vi "Transition State.vi"(8 "Error In":errorcluster, 10 "L       E \nIndicator":T1 caption="L      E", 11 "Present  State":T2) -> (0 "Error Out":errorcluster, 3 "Next State":T2)   [LabVIEW 2023]
doc: "This VI uses the present state and thre inputs L and E to determine the next state."
uses:
  controls/enum defining states.ctl
  controls/Boolean L E indictaor.ctl
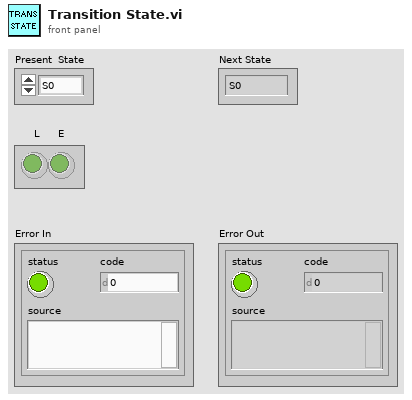
[diagram p1: front panel]
types:
  T1 = typedef "Boolean L E indictaor.ctl" = bool[]
  T2 = typedef "enum defining states.ctl" = enum16{"S0", "S1", "S2", "S3"}
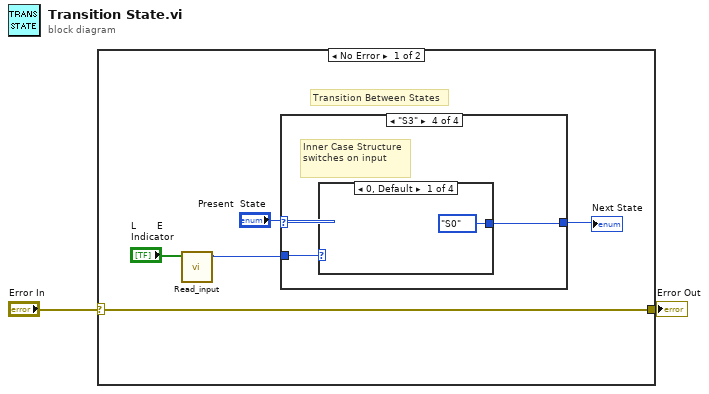
[diagram p0: block diagram]
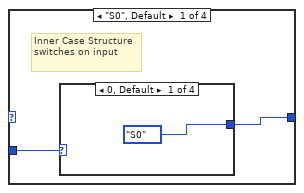
[diagram p2: hidden frame]
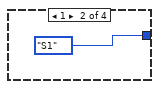
[diagram p3: hidden frame]
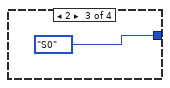
[diagram p4: hidden frame]
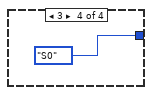
[diagram p5: hidden frame]
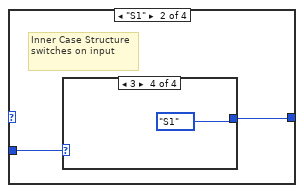
[diagram p6: hidden frame]
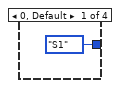
[diagram p7: hidden frame]
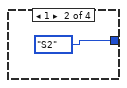
[diagram p8: hidden frame]
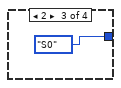
[diagram p9: hidden frame]
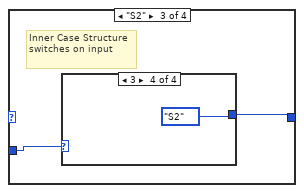
[diagram p10: hidden frame]
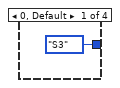
[diagram p11: hidden frame]
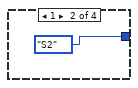
[diagram p12: hidden frame]
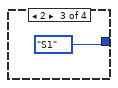
[diagram p13: hidden frame]
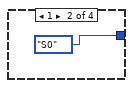
[diagram p14: hidden frame]
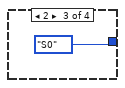
[diagram p15: hidden frame]
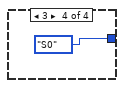
[diagram p16: hidden frame]
diagram:
  n1 = case shown="No Error" "Error In" {
    selector: "Error In" -> [w6 w32]
    tunnel: [w6 w32] -> w1
    frame No Error {
      # "Transition Between States"
      n2 = call "Read_input.vi"("L       E \nIndicator"="L       E \nIndicator") -> ("Input"=w3:u16)  [unwired: 10 in]
      n3 = case shown="\"S3\"" "Present  State" {
        tunnel: [w9 w15 w21 w27] -> w5
        tunnel: w3 -> [w8 w14 w20 w26]
        frame "S0", Default {
          # "Inner Case Structure\nswitches on input"
          n4 = case shown="0, Default" w8 {
            tunnel: [enum_defining_states."S0" ("State Enum") enum_defining_states."S1" ("State Enum") enum_defining_states."S0" ("State Enum") enum_defining_states."S0" ("State Enum")] -> w9
            frame 0, Default {
            }
            frame 1 {
            }
            frame 2 {
            }
            frame 3 {
            }
          }
        }
        frame "S1" {
          # "Inner Case Structure\nswitches on input"
          n5 = case shown="3" w14 {
            tunnel: [enum_defining_states."S1" ("State Enum") enum_defining_states."S2" ("State Enum") enum_defining_states."S0" ("State Enum") enum_defining_states."S1" ("State Enum")] -> w15
            frame 0, Default {
            }
            frame 1 {
            }
            frame 2 {
            }
            frame 3 {
            }
          }
        }
        frame "S2" {
          # "Inner Case Structure\nswitches on input"
          n6 = case shown="3" w20 {
            tunnel: [enum_defining_states."S3" ("State Enum") enum_defining_states."S2" ("State Enum") enum_defining_states."S1" ("State Enum") enum_defining_states."S2" ("State Enum")] -> w21
            frame 0, Default {
            }
            frame 1 {
            }
            frame 2 {
            }
            frame 3 {
            }
          }
        }
        frame "S3" {
          # "Inner Case Structure\nswitches on input"
          n7 = case shown="0, Default" w26 {
            tunnel: [enum_defining_states."S0" ("State Enum") enum_defining_states."S0" ("State Enum") enum_defining_states."S0" ("State Enum") enum_defining_states."S0" ("State Enum")] -> w27
            frame 0, Default {
            }
            frame 1 {
            }
            frame 2 {
            }
            frame 3 {
            }
          }
        }
      }
      "Next State" <- w5
    }
    frame Error {
    }
  }
  "Error Out" <- w1
